vi "ConfigureSupply.vi"(8 "error in (no error)":errorcluster, 9 "NoiseFrequency/Hz":i32[](array[numeric]) min=6 max=3000, 10 "Use Noise Rejecting":bool, 11 "Einstellungen":T1={"Channel Name"="1", "Source Delay (Sec)"=1.0, "Measurement:Sense"=1008, "voltage level"=0.0, "voltage level range"=20.0, "current limit"=0.02, "current limit range"=0.02, "resource name"="SUPPLY1"} {"current limit range" format="%_6p"; "current limit" format="%_6p"; "voltage level range" format="%_6p"; "voltage level" format="%_6p"; "Measurement:Sense" items=["Local"=1008, "Remote"=1009]; "Source Delay (Sec)" format="%_6p"}) -> (0 "error out":errorcluster, 3 "instrument handle out":refnum<k15>)   [LabVIEW 2018]
uses:
  Type/SupplyConfig.ctl
  <instrlib>/niDCPower/nidcpower.llb/niDCPower Source Mode.ctl
panel:
  # "Einstellungen"
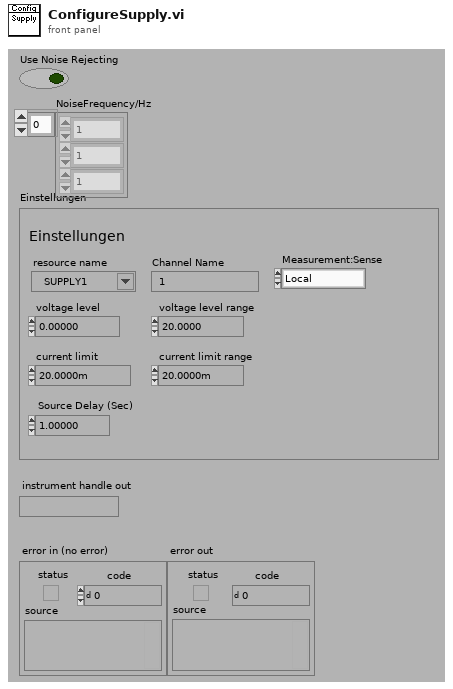
[diagram p1: front panel]
types:
  T1 = typedef "SupplyConfig.ctl" = cluster{"Channel Name":string, "Source Delay (Sec)":dbl, "Measurement:Sense":i32, "voltage level":dbl, "voltage level range":dbl, "current limit":dbl, "current limit range":dbl, "resource name":refnum<k15>}
  T2 = typedef "niDCPower Source Mode.ctl" = i32
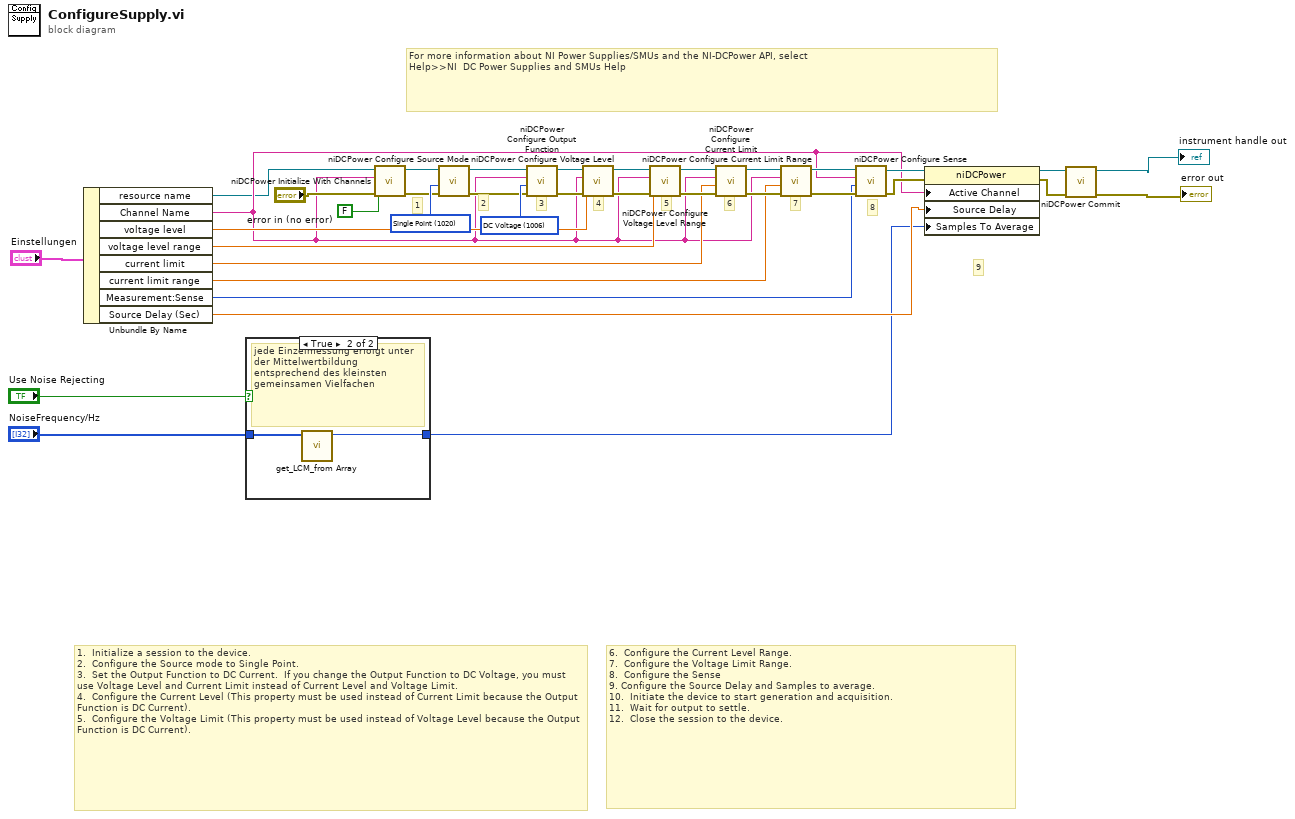
[diagram p0: block diagram]
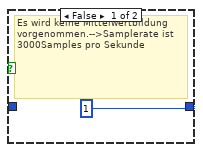
[diagram p2: hidden frame]
diagram:
  w33 = T2 1020 items=["Single Point"=1020, "Sequence"=1021] ("source mode")
  w36 = 1006 items=["DC Voltage"=1006, "DC Current"=1007] ("output function")
  # "8"
  # "For more information about NI Power Supplies/SMUs and the NI-DCPower API, select\nHelp>>NI  DC Power Supplies and SMUs Help"
  # "9"
  # "7"
  # "6"
  # "2"
  # "1.  Initialize a session to the device.\n2.  Configure the Source mode to Single Point.\n3.  Set the Output Function to DC Current.  If you change the Output Function to DC Voltage, you must use Voltage Level and Current Limit instead of Current Level and Voltage Limit.\n4.  Configure the Current Level (This property must be used instead of Current Limit because the Output Function is DC Current).\n5.  Configure the Voltage Limit (This property must be used instead of Voltage Level because the Output Function is DC Current)."
  # "3"
  # "6.  Configure the Current Level Range.\n7.  Configure the Voltage Limit Range.\n8.  Configure the Sense \n9. Configure the Source Delay and Samples to average.\n10.  Initiate the device to start generation and acquisition.\n11.  Wait for output to settle.\n12.  Close the session to the device."
  # "5"
  # "4"
  # "1"
  n1 = Unbundle By Name("Einstellungen") -> ("resource name"=w5:refnum<k15>, "Channel Name"=w8:string, "voltage level"=w14:dbl, "voltage level range"=w13:dbl, "current limit"=w12:dbl, "current limit range"=w11:dbl, "Measurement:Sense"=w10:i32, "Source Delay (Sec)"=w9:dbl)
  n2 = case shown="True" "Use Noise Rejecting" {
    tunnel: "NoiseFrequency/Hz" -> [_ w39]
    tunnel: [1 ("Measurement:Samples To Average") w38] -> w1
    frame False {
      # "Es wird keine Mittelwertbildung vorgenommen.-->Samplerate ist 3000Samples pro Sekunde"
    }
    frame True {
      # "jede Einzelmessung erfolgt unter der Mittelwertbildung entsprechend des kleinsten gemeinsamen Vielfachen"
      n3 = call "get_LCM_from Array.vi"("NoiseFrequency/Hz"=w39) -> ("lcm(x,y)"=w38:i64)  [unwired: 10 in]
    }
  }
  n4 = call <instrlib>:"niDCPower Initialize With Channels.vi"("error in (no error)"="error in (no error)", "reset (false)"=FALSE, "channels"=w8, "resource name"=w5) -> ("error out"=w31:errorcluster, "instrument handle out"=w32:refnum<k15>)  [unwired: 1 in, 5 out]
  n5 = call <instrlib>:"niDCPower Configure Source Mode.vi"("error in (no error)"=w31, "source mode"=w33, "instrument handle"=w32) -> ("error out"=w35:errorcluster, "instrument handle out"=w34:refnum<k15>)  [unwired: 7 out]
  n6 = call <instrlib>:"niDCPower Configure Output Function.vi"("error in (no error)"=w35, "output function"=w36, "channel name"=w8, "instrument handle"=w34) -> ("error out"=w23:errorcluster, "instrument handle out"=w24:refnum<k15>)  [unwired: 6 out]
  n7 = call <instrlib>:"niDCPower Configure Voltage Level.vi"("error in (no error)"=w23, "voltage level"=w14, "channel name"=w8, "instrument handle"=w24) -> ("error out"=w21:errorcluster, "instrument handle out"=w22:refnum<k15>)  [unwired: 6 in]
  n8 = call <instrlib>:"niDCPower Configure Voltage Level Range.vi"("error in (no error)"=w21, "voltage level range"=w13, "channel name"=w8, "instrument handle"=w22) -> ("error out"=w19:errorcluster, "instrument handle out"=w20:refnum<k15>)  [unwired: 6 in]
  n9 = call <instrlib>:"niDCPower Configure Current Limit.vi"("error in (no error)"=w19, "current limit"=w12, "channel name"=w8, "instrument handle"=w20) -> ("error out"=w17:errorcluster, "instrument handle out"=w18:refnum<k15>)  [unwired: 6 in]
  n10 = call <instrlib>:"niDCPower Configure Current Limit Range.vi"("error in (no error)"=w17, "current limit range"=w11, "channel name"=w8, "instrument handle"=w18) -> ("error out"=w15:errorcluster, "instrument handle out"=w16:refnum<k15>)  [unwired: 6 in]
  n11 = call <instrlib>:"niDCPower Configure Sense.vi"("error in (no error)"=w15, "sense"=w10, "channel name"=w8, "instrument handle"=w16) -> ("error out"=w30:errorcluster, "instrument handle out"=w29:refnum<k15>)  [unwired: 6 in]
  n12 = property class="niDCPower"(reference=w29, error in=w30, "Active Channel"=w8, "Source Delay"=w9, "Samples To Average"=w1) -> (reference out=w28:refnum<k15>, error out=w27:errorcluster)
  n13 = call <instrlib>:"niDCPower Commit.vi"("error in (no error)"=w27, "instrument handle"=w28) -> ("error out"=→"error out":errorcluster, "instrument handle out"=→"instrument handle out":refnum<k15>)  [unwired: 8 out]
